vi "7b_Boolean_Case(170382,170307).vi"() -> ()   [LabVIEW 2015]
panel:
  in  "stop":bool
  in  "Boolean":bool
  out "Output":dbl format="%.2f"
  in  "B":dbl format="%.2f"
  in  "A":dbl format="%.2f"
  # "Do not run this in continuous mode"
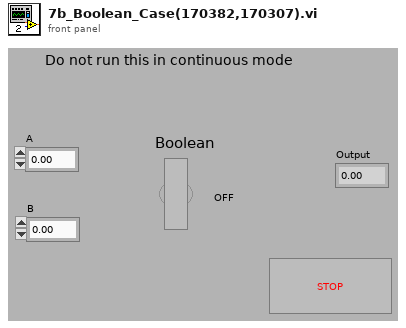
[diagram p1: front panel]
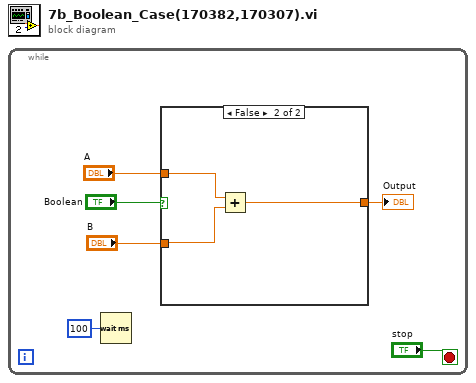
[diagram p0: block diagram]
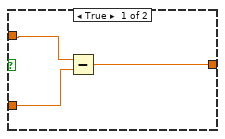
[diagram p2: hidden frame]
diagram:
  n1 = while {
    stop <- "stop" stop-if-true
    n2 = Wait (ms)(milliseconds to wait=u32 100) -> ()  [unwired: 1 out]
    n3 = case shown="False" "Boolean" {
      tunnel: "B" -> [w8 w11]
      tunnel: "A" -> [w9 w12]
      tunnel: [w7 w10] -> w4
      frame True {
        n4 = Subtract(x=w9, y=w8) -> (x-y=w7:dbl)
      }
      frame False {
        n5 = Add(x=w12, y=w11) -> (x+y=w10:dbl)
      }
    }
    "Output" <- w4
  }
